vi "close_connection.vi"(1 "error in":errorcluster, 3 "VISA resource name out":refnum<visa-resource-name>) -> (0 "OUTPUT string":string)   [LabVIEW 2015]
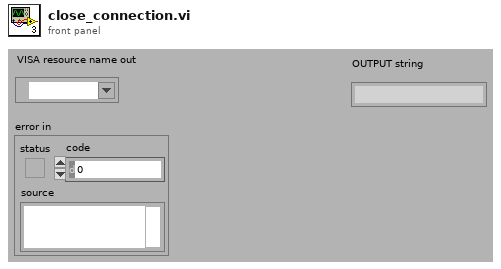
[diagram p1: front panel]
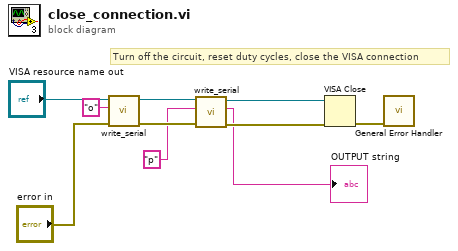
[diagram p0: block diagram]
diagram:
  # "Turn off the circuit, reset duty cycles, close the VISA connection"
  n1 = call "write_serial.vi"("error in (no error)"="error in", "write buffer"="o", "VISA resource name"="VISA resource name out") -> ("error out"=w5:errorcluster, "VISA resource name out"=w6:refnum<visa-resource-name>)  [unwired: 2 in, 1 out]
  n2 = call "write_serial.vi"("error in (no error)"=w5, "write buffer"="p", "VISA resource name"=w6) -> ("error out"=w4:errorcluster, "read buffer"=→"OUTPUT string":string, "VISA resource name out"=w3:refnum<visa-resource-name>)  [unwired: 2 in]
  n3 = VISA Close(VISA resource name=w3, error in (no error)=w4) -> (error out=w10:errorcluster)
  n4 = call <vilib>:"General Error Handler.vi"("error in (no error)"=w10) -> ()  [unwired: 10 in, 5 out]
